vi "PH_GUI.set boolean GUI object.vi"(0 "Caption":string, 1 "Visible (true)":bool=TRUE, 2 "Boolean Knob GUI Ref":refnum<vi>, 3 "Value":bool, 4 "Blinking? (false)":bool, 5 "error in (no error)":errorcluster, 7 "Tip Strip":string) -> (19 "error out":errorcluster)   [LabVIEW 2014, in "PH_Common.lvlib"]
doc: "Sets value and more for the referenced GUI object."
uses:
  PH_Common.lvlib
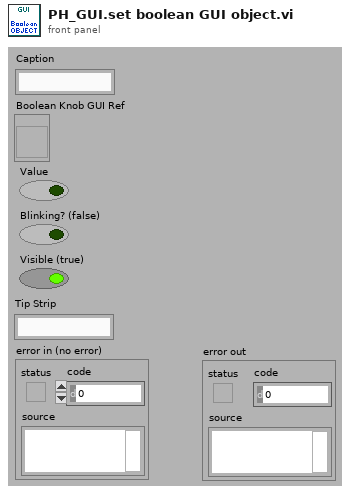
[diagram p1: front panel]
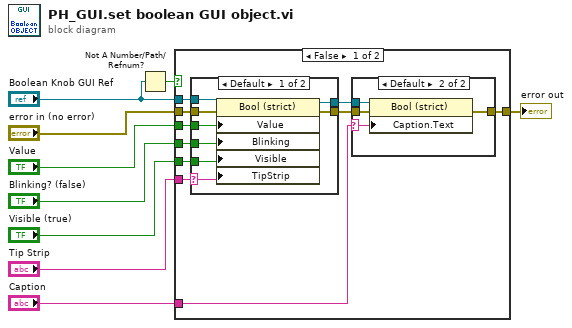
[diagram p0: block diagram]
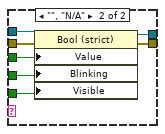
[diagram p3: hidden frame]
diagram:
  n1 = Not A Number/Path/Refnum?(number/path/refnum="Boolean Knob GUI Ref") -> (NaN/Path/Refnum?=w9:bool)
  n2 = case shown="False" w9 {
    tunnel: "Boolean Knob GUI Ref" -> [w19 _]
    tunnel: "Value" -> [w18 _]
    tunnel: "error in (no error)" -> [w17 w40]
    tunnel: [w13 w40] -> w7
    tunnel: "Blinking? (false)" -> [w16 _]
    tunnel: "Visible (true)" -> [w15 _]
    tunnel: "Tip Strip" -> [w14 _]
    tunnel: "Caption" -> [w10 _]
    frame False {
      n3 = case shown="Default" w14 {
        selector: w14 -> [w26 _]
        tunnel: w19 -> [w32 w39]
        tunnel: w18 -> [w31 w38]
        tunnel: w17 -> [w30 w37]
        tunnel: [w29 w36] -> w12
        tunnel: w16 -> [w28 w35]
        tunnel: w15 -> [w27 w34]
        tunnel: [w25 w33] -> w11
        frame Default {
          n4 = property class="Bool (strict)"(reference=w32, error in=w30, "Value"=w31, "Blinking"=w28, "Visible"=w27, "TipStrip"=w26) -> (reference out=w25:refnum<vi>, error out=w29:errorcluster)
        }
        frame "", "N/A" {
          n5 = property class="Bool (strict)"(reference=w39, error in=w37, "Value"=w38, "Blinking"=w35, "Visible"=w34) -> (reference out=w33:refnum<vi>, error out=w36:errorcluster)
        }
      }
      n6 = case shown="Default" w10 {
        selector: w10 -> [_ w21]
        tunnel: [w20 w24] -> w13
        tunnel: w12 -> [w20 w23]
        tunnel: w11 -> [_ w22]
        frame "", "N/A" {
        }
        frame Default {
          n7 = property class="Bool (strict)"(reference=w22, error in=w23, "Caption.Text"=w21) -> (error out=w24:errorcluster)  [unwired: 1 out]
        }
      }
    }
    frame True {
    }
  }
  "error out" <- w7
